vi "AFG Points Gen.vi"(0 "Delay":dbl=50.0, 1 "Spacing":dbl=50.0, 2 "Set Pulse Conf":T1, 3 "Reset Pulse Conf":T1) -> (7 "Frequency":dbl, 8 "gain":dbl, 9 "Offset":dbl, 10 "Points Array":dbl[](array[numeric]))   [LabVIEW 2020, in "Actor_AFG.lvlib"]
uses:
  Actor_AFG.lvlib
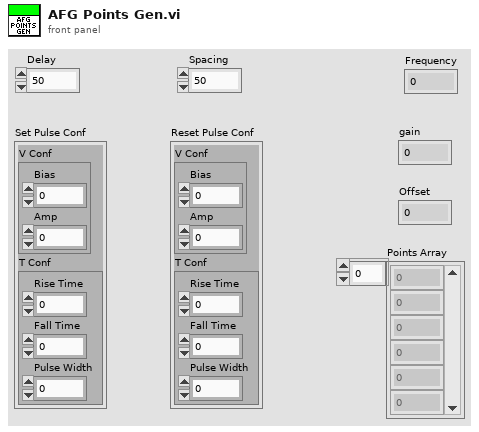
[diagram p1: front panel]
types:
  T1 = cluster{"V Conf":cluster{"Bias":dbl, "Amp":dbl}, "T Conf":cluster{"Rise Time":dbl, "Fall Time":dbl, "Pulse Width":dbl}}
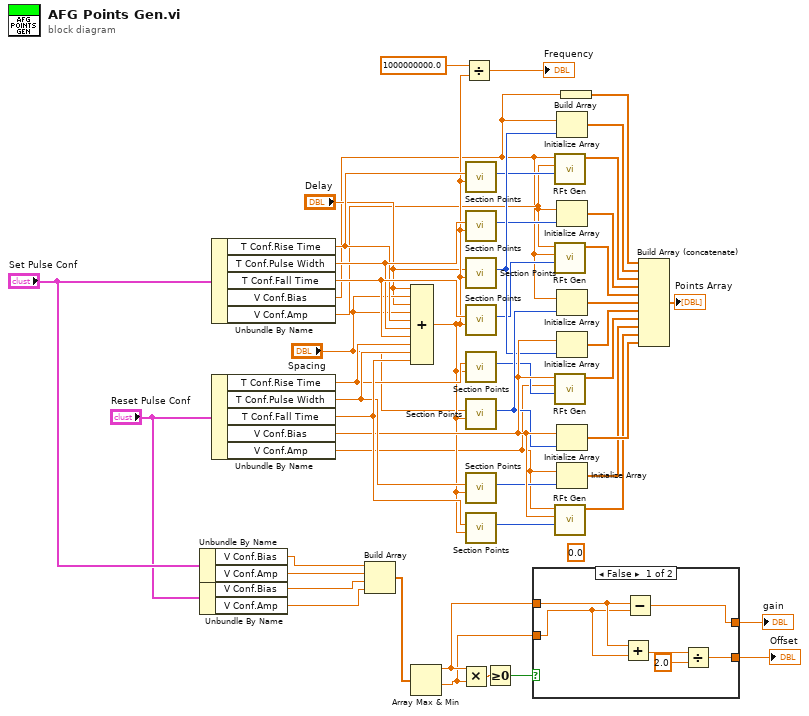
[diagram p0: block diagram]
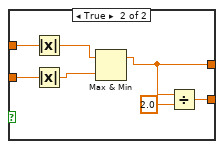
[diagram p2: hidden frame]
diagram:
  (unwired) 0.0 ("element")
  n1 = Unbundle By Name("Set Pulse Conf") -> ("V Conf.Bias"=w8:dbl, "V Conf.Amp"=w7:dbl)
  n2 = Unbundle By Name("Reset Pulse Conf") -> ("V Conf.Bias"=w6:dbl, "V Conf.Amp"=w5:dbl)
  n3 = Unbundle By Name("Set Pulse Conf") -> ("T Conf.Rise Time"=w41:dbl, "T Conf.Pulse Width"=w42:dbl, "T Conf.Fall Time"=w43:dbl, "V Conf.Bias"=w1:dbl, "V Conf.Amp"=w13:dbl)
  n4 = Unbundle By Name("Reset Pulse Conf") -> ("T Conf.Rise Time"=w45:dbl, "T Conf.Pulse Width"=w46:dbl, "T Conf.Fall Time"=w47:dbl, "V Conf.Bias"=w44:dbl, "V Conf.Amp"=w12:dbl)
  n5 = Build Array(w8, w7, w6, w5) -> (w4:dbl[])
  n6 = Compound Arithmetic op=ADD("Delay", "Spacing", "Delay", "Spacing", w41, w42, w43, w45, w46, w47) -> (w37:dbl)
  n7 = Array Max & Min(array=w4) -> (max value=w3:dbl, min value=w2:dbl)  [unwired: 2 out]
  n8 = Multiply(x=w3, y=w2) -> (x*y=w16:dbl)
  n9 = Divide(x=1000000000.0, y=w37) -> (x/y=→"Frequency":dbl)
  n10 = call "Section Points.vi"("Period"=w37, "Delay"=w41) -> ("Seciton Points"=w28:u16)  [unwired: 9 in]
  n11 = call "Section Points.vi"("Period"=w37, "Delay"=w42) -> ("Seciton Points"=w29:u16)  [unwired: 9 in]
  n12 = call "Section Points.vi"("Period"=w37, "Delay"="Delay") -> ("Seciton Points"=w39:u16)  [unwired: 9 in]
  n13 = call "Section Points.vi"("Period"=w37, "Delay"=w43) -> ("Seciton Points"=w30:u16)  [unwired: 9 in]
  n14 = call "Section Points.vi"("Period"=w37, "Delay"=w45) -> ("Seciton Points"=w31:u16)  [unwired: 9 in]
  n15 = call "Section Points.vi"("Period"=w37, "Delay"="Spacing") -> ("Seciton Points"=w40:u16)  [unwired: 9 in]
  n16 = call "Section Points.vi"("Period"=w37, "Delay"=w46) -> ("Seciton Points"=w32:u16)  [unwired: 9 in]
  n17 = call "Section Points.vi"("Period"=w37, "Delay"=w47) -> ("Seciton Points"=w33:u16)  [unwired: 9 in]
  n18 = Greater Or Equal To 0?(x=w16) -> (x >= 0?=w15:bool)
  n19 = case shown="False" w15 {
    tunnel: [w51 w58] -> w14
    tunnel: [w52 w59] -> w11
    tunnel: w3 -> [w50 w56]
    tunnel: w2 -> [w49 w55]
    frame False {
      n20 = Add(x=w50, y=w49) -> (x+y=w54:dbl)
      n21 = Subtract(x=w50, y=w49) -> (x-y=w51:dbl)
      n22 = Divide(x=w54, y=2.0) -> (x/y=w52:dbl)
    }
    frame True {
      n23 = Absolute Value(x=w56) -> (abs(x)=w61:dbl)
      n24 = Absolute Value(x=w55) -> (abs(x)=w60:dbl)
      n25 = Max & Min(x=w61, y=w60) -> (max(x,y)=w58:dbl)  [unwired: 1 out]
      n26 = Divide(x=w58, y=2.0) -> (x/y=w59:dbl)
    }
  }
  "gain" <- w14
  "Offset" <- w11
  n27 = call "RFt Gen.vi"("Seciton Num"=w28, "End V"=w13, "Start V"=w1) -> ("Points"=w19:dbl[])  [unwired: 8 in]
  n28 = call "RFt Gen.vi"("Seciton Num"=w30, "End V"=w1, "Start V"=w13) -> ("Points"=w21:dbl[])  [unwired: 8 in]
  n29 = call "RFt Gen.vi"("Seciton Num"=w31, "End V"=w12, "Start V"=w44) -> ("Points"=w24:dbl[])  [unwired: 8 in]
  n30 = call "RFt Gen.vi"("Seciton Num"=w33, "End V"=w44, "Start V"=w12) -> ("Points"=w26:dbl[])  [unwired: 8 in]
  n31 = Initialize Array(w1, w39) -> (w18:dbl[])
  n32 = Initialize Array(w13, w29) -> (w20:dbl[])
  n33 = Initialize Array(w1, w40) -> (w22:dbl[])
  n34 = Initialize Array(w44, w39) -> (w23:dbl[])
  n35 = Initialize Array(w44, w40) -> (w27:dbl[])
  n36 = Initialize Array(w12, w32) -> (w25:dbl[])
  n37 = Build Array(w1) -> (w17:dbl[])
  n38 = Build Array (concatenate)(w17, w18, w19, w20, w21, w22, w23, w24, w25, w26, w27) -> (→"Points Array":dbl[])
